vi "reset.vi"(8 "error in (no error)":errorcluster, 11 "IntrinsicImagingMG091001 in":refnum<class "DataCollectionMG091001IntrinsicImaging.lvclass">) -> (0 "error out":errorcluster, 3 "IntrinsicImagingMG091001 out":refnum<class "DataCollectionMG091001IntrinsicImaging.lvclass">)   [LabVIEW 2010, in "DataCollectionMG091001IntrinsicImaging.lvclass"]
uses:
  DataCollectionMG091001IntrinsicImaging.lvclass
  common/classes/ImageCollection/ImageCollection/ImageCollection.lvclass
  DataCollectionMG091001IntrinsicImaging.lvclass/DataCollectionMG091001IntrinsicImaging.ctl
  common/classes/ErrorController/ErrorController/class_data.vi
  common/classes/ErrorController/ErrorController/ErrorController.lvclass
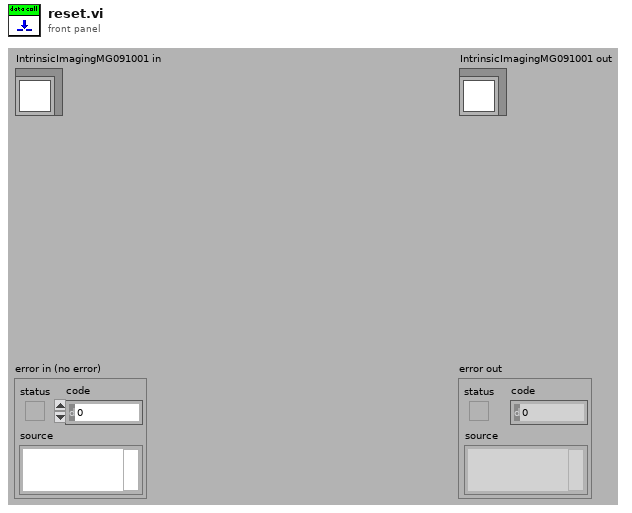
[diagram p1: front panel]
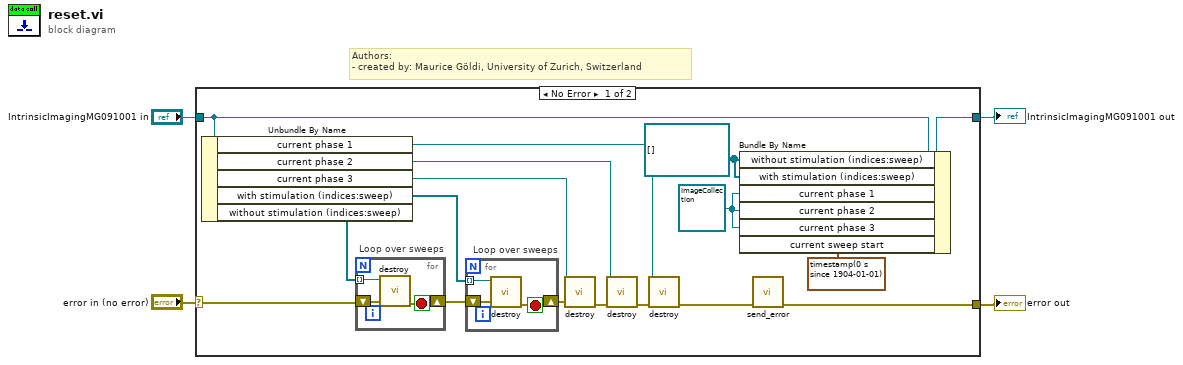
[diagram p0: block diagram]
diagram:
  # "Authors: \n- created by: Maurice Göldi, University of Zurich, Switzerland"
  n1 = case shown="No Error" "error in (no error)" {
    selector: "error in (no error)" -> [w14 w28]
    tunnel: "IntrinsicImagingMG091001 in" -> [w16 w29]
    tunnel: [w15 w29] -> w3
    tunnel: [w6 w28] -> w1
    frame No Error {
      w8 = refnum<class "ImageCollection.lvclass"> refnum ("ImageCollection.lvclass")
      w13 = refnum<class "ImageCollection.lvclass">[] []
      n2 = Unbundle By Name(w16) -> ("current phase 1"=w9:refnum<class "ImageCollection.lvclass">, "current phase 2"=w10:refnum<class "ImageCollection.lvclass">, "current phase 3"=w19:refnum<class "ImageCollection.lvclass">, "with stimulation (indices:sweep)"=w20:refnum<class "ImageCollection.lvclass">[], "without stimulation (indices:sweep)"=w21:refnum<class "ImageCollection.lvclass">[])
      n3 = for "Loop over sweeps" {
        tunnel: w21 -> [w27] mode=indexing
        shift-right: [w25] -> w18
        shift-left: w14 -> [w26]
        stop <- w25 stop-if-true
        n4 = call-dynamic "destroy.vi"("error in (no error)"=w26, "ImageCollection in"=w27) -> ("error out"=w25:errorcluster)  [unwired: 8 in, 1 out]
      }
      n5 = for "Loop over sweeps" {
        tunnel: w20 -> [w24] mode=indexing
        shift-right: [w22] -> w17
        shift-left: w18 -> [w23]
        stop <- w22 stop-if-true
        n6 = call-dynamic "destroy.vi"("error in (no error)"=w23, "ImageCollection in"=w24) -> ("error out"=w22:errorcluster)  [unwired: 8 in, 1 out]
      }
      n7 = call-dynamic "destroy.vi"("error in (no error)"=w17, "ImageCollection in"=w19) -> ("error out"=w11:errorcluster)  [unwired: 8 in, 1 out]
      n8 = call-dynamic "destroy.vi"("error in (no error)"=w11, "ImageCollection in"=w10) -> ("error out"=w12:errorcluster)  [unwired: 8 in, 1 out]
      n9 = call-dynamic "destroy.vi"("error in (no error)"=w12, "ImageCollection in"=w9) -> ("error out"=w7:errorcluster)  [unwired: 8 in, 1 out]
      n10 = Bundle By Name(cluster=w16, "without stimulation (indices:sweep)"=w13, "with stimulation (indices:sweep)"=w13, "current phase 1"=w8, "current phase 2"=w8, "current phase 3"=w8, "current sweep start"=timestamp(0 s since 1904-01-01) ("current data.current sweep start")) -> (w15:refnum<class "DataCollectionMG091001IntrinsicImaging.lvclass">)
      n11 = call "send_error.vi"("error in (no error)"=w7) -> ("error out"=w6:errorcluster)  [unwired: 10 in]
    }
    frame Error {
    }
  }
  "error out" <- w1
  "IntrinsicImagingMG091001 out" <- w3
